vi "HW_GEN - Data Queue Manage FGV.vi"(7 "Oper.":T2=enum."Add Chan", 8 "error in":errorcluster, 10 "ChanTag":string, 11 "Add Chan":T1) -> (0 "error out":errorcluster, 2 "ChanInfo":cluster{"Queue Name":string, "index":i32})   [LabVIEW 2016]
uses:
  Ctrls/HardWare _ Data Queue Manage FGV Operation.ctl
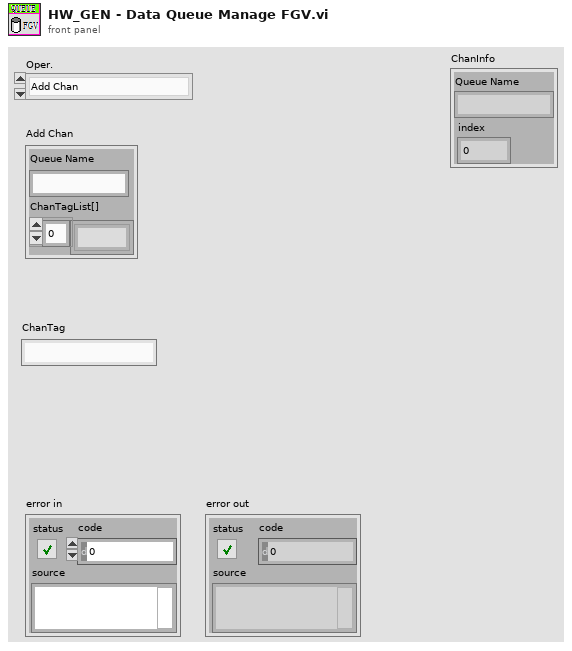
[diagram p1: front panel]
types:
  T1 = cluster{"Queue Name":string, "ChanTagList[]":string[]}
  T2 = typedef "HardWare _ Data Queue Manage FGV Operation.ctl" = enum16{"Initialize", "Add Chan", "Read Chan"}
  T3 = cluster{"Queue Name":string, "ChanTagList[]":string[]}[]
  T4 = cluster{"Queue Name":string, "index of element":i32}
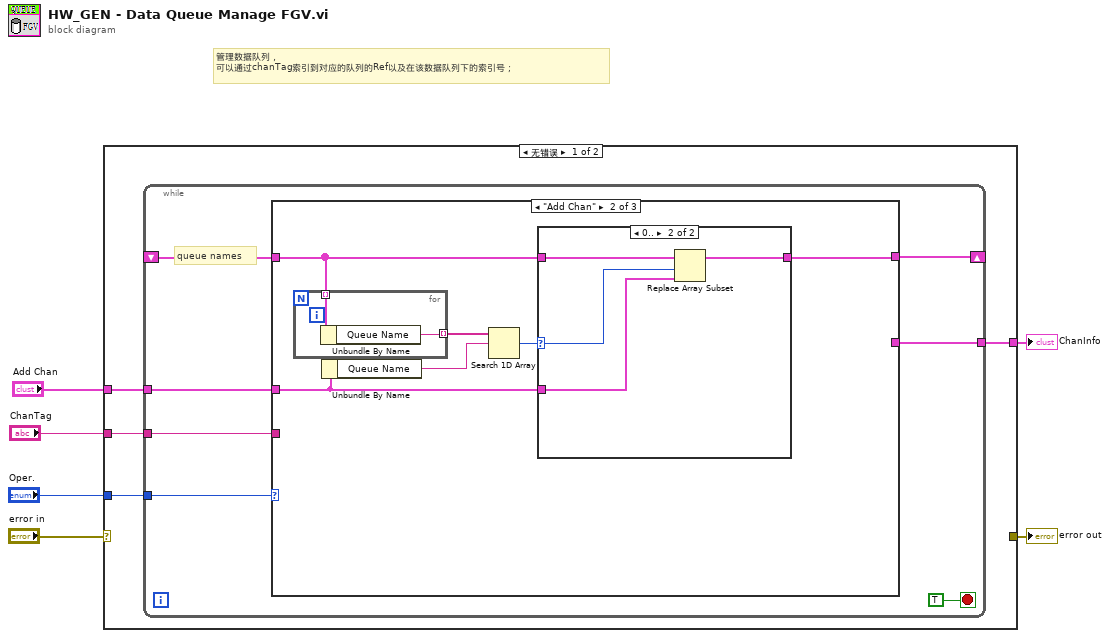
[diagram p0: block diagram]
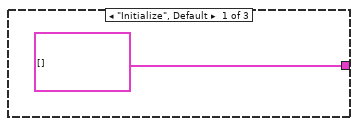
[diagram p2: hidden frame]
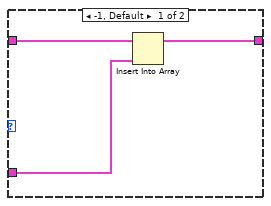
[diagram p3: hidden frame]
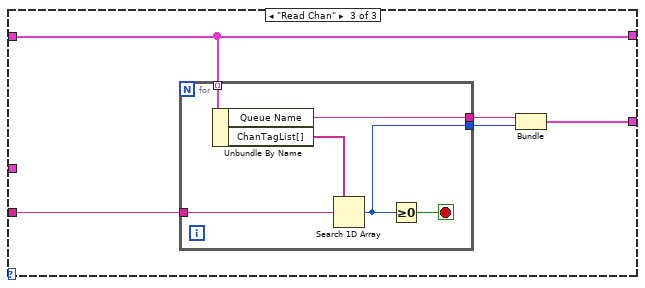
[diagram p4: hidden frame]
diagram:
  # "管理数据队列，\n可以通过chanTag索引到对应的队列的Ref以及在该数据队列下的索引号；"
  n1 = case shown="无错误" "error in" {
    selector: "error in" -> [_ w45]
    tunnel: [_ w45] -> w5
    tunnel: "Oper." -> [w10 _]
    tunnel: "Add Chan" -> [w9 _]
    tunnel: "ChanTag" -> [w8 _]
    tunnel: [w7 _] -> w1
    frame No Error {
      n2 = while {
        tunnel: w10 -> [w16]
        tunnel: w9 -> [w15]
        tunnel: w8 -> [w14]
        shift-right: [w13] -> _
        shift-left: _ -> [w12]
        tunnel: [w11] -> w7
        stop <- TRUE stop-if-true
        # "queue names"
        n3 = case shown="\"Add Chan\"" w16 {
          tunnel: w15 -> [_ w19 _]
          tunnel: w14 -> [_ _ w38]
          tunnel: [T3 [] w20 w37] -> w13
          tunnel: w12 -> [_ w21 w37]
          tunnel: [_ _ w34] -> w11
          frame "Initialize", Default {
          }
          frame "Add Chan" {
            n4 = for {
              tunnel: w21 -> [w33] mode=indexing
              tunnel: [w32] -> w24 mode=indexing
              n5 = Unbundle By Name(w33) -> ("Queue Name"=w32:string)
            }
            n6 = Unbundle By Name(w19) -> ("Queue Name"=w23:string)
            n7 = Search 1D Array(1D array=w24, element=w23) -> (index of element=w22:i32)  [unwired: 1 in]
            n8 = case shown="0.." w22 {
              selector: w22 -> [_ w29]
              tunnel: w21 -> [w27 w31]
              tunnel: [w26 w30] -> w20
              tunnel: w19 -> [w25 w28]
              frame -1, Default {
                n9 = Insert Into Array(array=w27, new element=w25) -> (w26:T3)  [unwired: 1 in]
              }
              frame 0.. {
                n10 = Replace Array Subset(array=w31, new element=w28, index=w29) -> (w30:T3)
              }
            }
          }
          frame "Read Chan" {
            n11 = for {
              tunnel: w37 -> [w44] mode=indexing
              tunnel: w38 -> [w42]
              tunnel: [w40] -> w36
              tunnel: [w39] -> w35
              stop <- w41 stop-if-true
              n12 = Unbundle By Name(w44) -> ("Queue Name"=w40:string, "ChanTagList[]"=w43:string[])
              n13 = Search 1D Array(1D array=w43, element=w42) -> (index of element=w39:i32)  [unwired: 1 in]
              n14 = Greater Or Equal To 0?(x=w39) -> (x >= 0?=w41:bool)
            }
            n15 = Bundle("Queue Name"=w36, "index of element"=w35) -> (w34:T4)  [unwired: 1 in]
          }
        }
      }
    }
    frame Error {
    }
  }
  "error out" <- w5
  "ChanInfo" <- w1
